vi "U6 Multiple IO Example Loop.vi"() -> ()   [LabVIEW 2021]
panel:
  in  "Interval (ms)":u32=500
  in  "stop":bool
  out "Read Values":T1 {"AIN3" format="%.6f"; "AIN2" format="%.6f"; "AIN1" format="%.6f"; "AIN0" format="%.6f"}
  in  "Write Values":T2 {"DAC1" format="%.4f"; "DAC0" format="%.4f"}
  out "Error Message":string
  in  "error in":errorcluster
  out "error out":errorcluster
  # "Outputs DAC0-DAC1 and FIO2-FIO3.  Aquires AIN0-AIN3 and FIO0-FIO1.  Uses USB on the first found U6.\n\nThis uses the LabVIEW utility AddS-Go-Get.vi, rather than calling eAddGoGet from the UD driver.  The utility\nVI has better/easier error handling and is normally preferred, but eAddGoGet is a single call to the UD driver\nso often preferred if you will have parallel driver calls to the same handle within the same thread (none of\nour examples do this)."
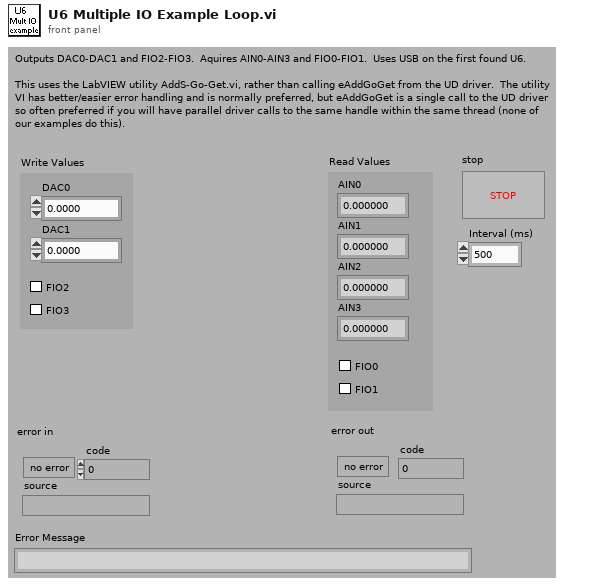
[diagram p1: front panel]
types:
  T1 = cluster{"AIN0":dbl, "AIN1":dbl, "AIN2":dbl, "AIN3":dbl, "FIO0":bool, "FIO1":bool}
  T2 = cluster{"DAC0":dbl, "DAC1":dbl, "FIO2":bool, "FIO3":bool}
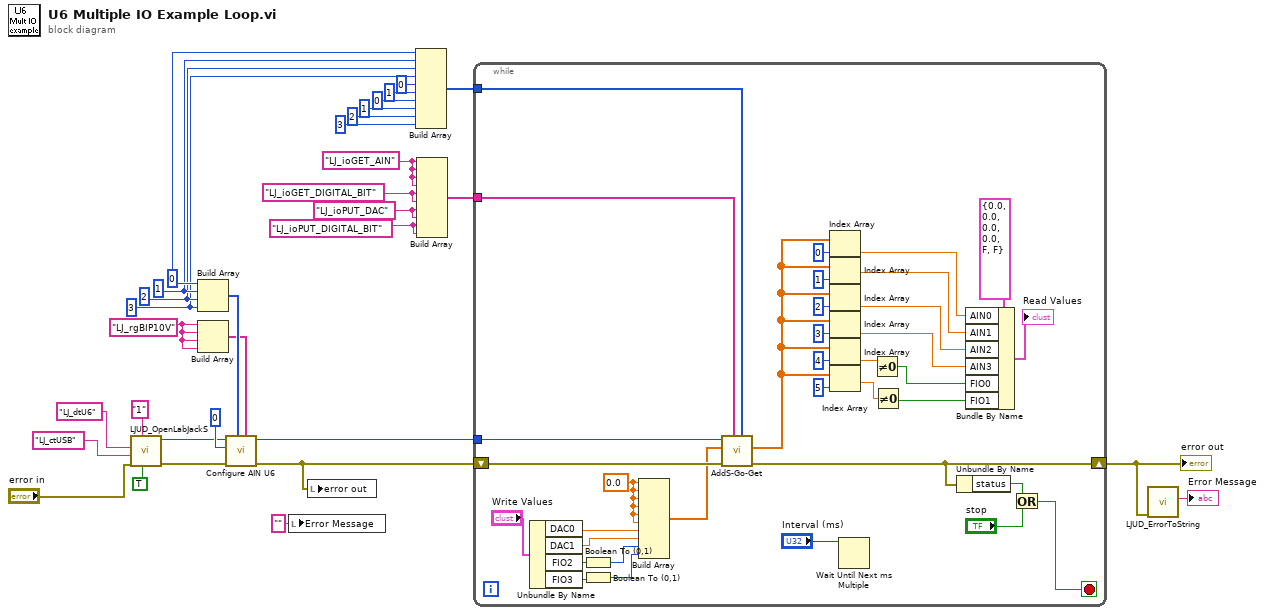
[diagram p0: block diagram]
diagram:
  w24 = "LJ_ioPUT_DIGITAL_BIT" ("IOType")
  w25 = "LJ_ioPUT_DAC" ("IOType")
  w27 = "LJ_ioGET_AIN" ("IOType")
  w20 = 3 ("SettlingFactor")
  w21 = 2 ("SettlingFactor")
  w22 = 1 ("SettlingFactor")
  w23 = 0 ("SettlingFactor")
  w9 = "LJ_rgBIP10V" ("AIN Range")
  w26 = "LJ_ioGET_DIGITAL_BIT" ("IOType")
  n1 = call "LJUD_OpenLabJackS.vi"("FirstFound"=TRUE, "Address"="1", "error in"="error in", "ConnectionType"="LJ_ctUSB", "DeviceType"="LJ_dtU6") -> ("error out"=w11:errorcluster, "Handle"=w7:i32)  [unwired: 4 in, 1 out]
  n2 = Build Array(w23, w22, w21, w20) -> (w10:i32[])
  n3 = Build Array(w9, w9, w9, w9) -> (w8:string[])
  n4 = call "Configure AIN U6.vi"("Ranges"=w8, "Positive Channels"=w10, "error in"=w11, "Resolution"=0, "Handle In"=w7) -> ("error out"=w2:errorcluster, "Handle Out"=w30:i32)  [unwired: 5 in]
  n5 = local write "Error Message"("" ("Error Message")) -> ()
  n6 = local write "error out"(w2) -> ()
  n7 = Build Array(w23, w22, w21, w20, 0 ("Input Element"), 1 ("Input Element"), 0 ("Input Element"), 1 ("Input Element"), 2 ("Input Element"), 3 ("Input Element")) -> (w12:i32[])
  n8 = Build Array(w27, w27, w27, w27, w26, w26, w25, w25, w24, w24) -> (w13:string[])
  n9 = while {
    tunnel: w30 -> [w67]
    tunnel: w13 -> [w65]
    tunnel: w12 -> [w64]
    shift-right: [w36] -> w29
    shift-left: w2 -> [w66]
    stop <- w33 stop-if-true
    w63 = 0.0 ("Input Element")
    n10 = Unbundle By Name("Write Values") -> ("DAC0"=w58:dbl, "DAC1"=w57:dbl, "FIO2"=w56:bool, "FIO3"=w55:bool)
    n11 = Boolean To (0,1)(Boolean=w56) -> (0, 1=w62:i16)
    n12 = Boolean To (0,1)(Boolean=w55) -> (0, 1=w61:i16)
    n13 = Build Array(w63, w63, w63, w63, w63, w63, w58, w57, w62, w61) -> (w60:dbl[])
    n14 = call "AddS-Go-Get.vi"("Channels"=w64, "IOTypes"=w65, "error in"=w66, "Values Write"=w60, "Handle In"=w67) -> ("error out"=w36:errorcluster, "Values Read"=w45:dbl[])  [unwired: 4 in, 1 out]
    n15 = Index Array(array=w45, index=0 ("Index")) -> (element=w43:dbl)
    n16 = Index Array(array=w45, index=1 ("Index")) -> (element=w42:dbl)
    n17 = Index Array(array=w45, index=2 ("Index")) -> (element=w41:dbl)
    n18 = Index Array(array=w45, index=3 ("Index")) -> (element=w40:dbl)
    n19 = Index Array(array=w45, index=4 ("Index")) -> (element=w39:dbl)
    n20 = Index Array(array=w45, index=5 ("Index")) -> (element=w38:dbl)
    n21 = Wait Until Next ms Multiple(millisecond multiple="Interval (ms)") -> ()  [unwired: 1 out]
    n22 = Not Equal To 0?(x=w39) -> (x != 0?=w51:bool)
    n23 = Not Equal To 0?(x=w38) -> (x != 0?=w52:bool)
    n24 = Unbundle By Name(w36) -> ("status"=w35:bool)
    n25 = Bundle By Name(cluster=T1 {"AIN0"=0.0, "AIN1"=0.0, "AIN2"=0.0, "AIN3"=0.0, "FIO0"=FALSE, "FIO1"=FALSE} ("Read Values"), "AIN0"=w43, "AIN1"=w42, "AIN2"=w41, "AIN3"=w40, "FIO0"=w51, "FIO1"=w52) -> (→"Read Values":T1)
    n26 = Or(x=w35, y="stop") -> (x .or. y?=w33:bool)
  }
  "error out" <- w29
  n27 = call "LJUD_ErrorToString.vi"("error in"=w29) -> ("String"=→"Error Message":string)  [unwired: 10 in]
